vi "Get Time.vi"() -> (3 "Time":string)   [LabVIEW 2015, in "Utility VIs.lvlib"]
uses:
  Utility VIs.lvlib
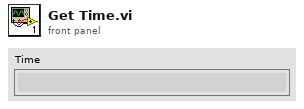
[diagram p1: front panel]
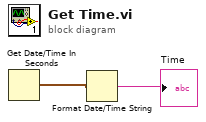
[diagram p0: block diagram]
diagram:
  n1 = Get Date/Time In Seconds() -> (seconds since 1Jan1904=w2:timestamp)
  n2 = Format Date/Time String(seconds (now)=w2) -> (date/time string=→"Time":string)  [unwired: 2 in]
